vi "MeanData.vi"(11 "Prop in":T1[](array[typedef])) -> (3 "Poperties out":T1={"Raw Data"=[[0.0], [0.0234375], [0.9609375]], "Poperties"={"RMS values"=[], "Max"=[], "Min"=[], "A(8)"=[], "t"=0.0, "A(8) Axis"=0.0, "Aw"=[], "Ak 30min"=0.0, "Ak_axis"=0, "Spec"=[]}, "Power Spectrum / PSD"=[]})   [LabVIEW 2019]
uses:
  Communication/TypeDef/#TypeDef_PropGraph.ctl
  Communication/TypeDef/#TypeDef_PropertiesToSave.ctl
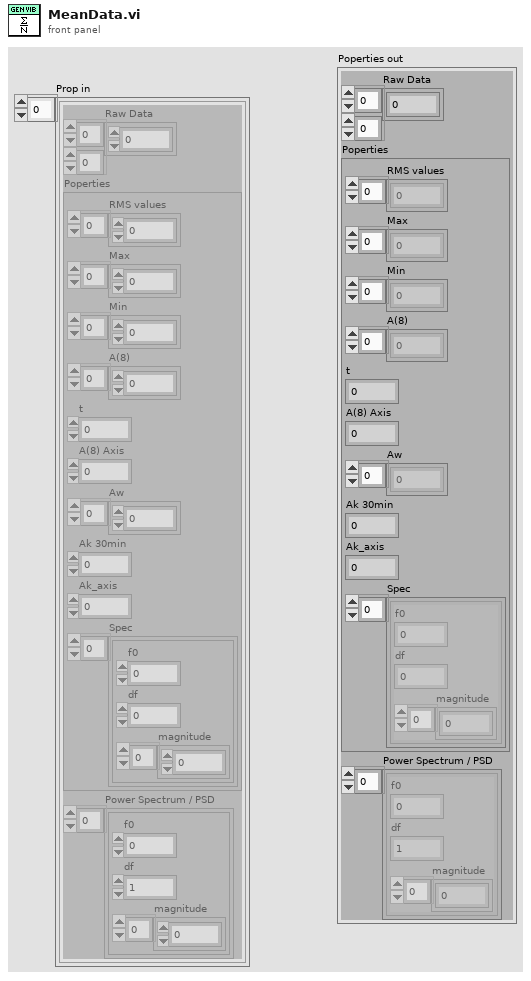
[diagram p1: front panel]
types:
  T1 = typedef "#TypeDef_PropGraph.ctl" = cluster{"Raw Data":dbl[][], "Poperties":T2, "Power Spectrum / PSD":cluster{"f0":dbl, "df":dbl, "magnitude":dbl[]}[]}
  T2 = typedef "#TypeDef_PropertiesToSave.ctl" = cluster{"RMS values":dbl[], "Max":dbl[], "Min":dbl[], "A(8)":dbl[], "t":dbl, "A(8) Axis":dbl, "Aw":dbl[], "Ak 30min":dbl, "Ak_axis":i32, "Spec":cluster{"f0":dbl, "df":dbl, "magnitude":dbl[]}[]}
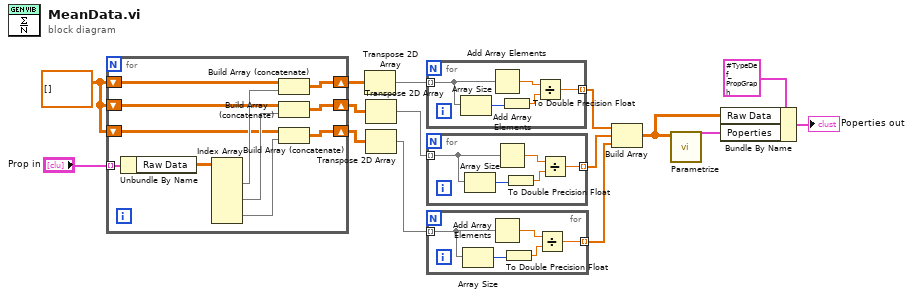
[diagram p0: block diagram]
diagram:
  w6 = dbl[][] []
  n1 = for {
    tunnel: "Prop in" -> [w26] mode=indexing
    shift-right: [w25] -> w7
    shift-left: w6 -> [w24]
    shift-right: [w20] -> w9
    shift-left: w6 -> [w19]
    shift-right: [w17] -> w11
    shift-left: w6 -> [w16]
    n2 = Unbundle By Name(w26) -> ("Raw Data"=w23:dbl[][])
    n3 = Index Array(array=w23) -> (element #1=w22:dbl[], element #2=w21:dbl[], element #3=w18:dbl[])  [unwired: 6 in]
    n4 = Build Array (concatenate)(w24, w22) -> (w25:dbl[][])
    n5 = Build Array (concatenate)(w19, w21) -> (w20:dbl[][])
    n6 = Build Array (concatenate)(w16, w18) -> (w17:dbl[][])
  }
  n7 = Transpose 2D Array(2D array=w7) -> (transposed array=w8:dbl[][])
  n8 = Transpose 2D Array(2D array=w9) -> (transposed array=w10:dbl[][])
  n9 = Transpose 2D Array(2D array=w11) -> (transposed array=w12:dbl[][])
  n10 = for {
    tunnel: w8 -> [w31] mode=indexing
    tunnel: [w30] -> w13 mode=indexing
    n11 = Array Size(array=w31) -> (size(s)=w29:i32)
    n12 = Add Array Elements(numeric array=w31) -> (sum=w28:dbl)
    n13 = To Double Precision Float(number=w29) -> (double precision float=w27:dbl)
    n14 = Divide(x=w28, y=w27) -> (x/y=w30:dbl)
  }
  n15 = for {
    tunnel: w10 -> [w36] mode=indexing
    tunnel: [w35] -> w14 mode=indexing
    n16 = Array Size(array=w36) -> (size(s)=w34:i32)
    n17 = Add Array Elements(numeric array=w36) -> (sum=w33:dbl)
    n18 = To Double Precision Float(number=w34) -> (double precision float=w32:dbl)
    n19 = Divide(x=w33, y=w32) -> (x/y=w35:dbl)
  }
  n20 = for {
    tunnel: w12 -> [w41] mode=indexing
    tunnel: [w40] -> w15 mode=indexing
    n21 = Array Size(array=w41) -> (size(s)=w39:i32)
    n22 = Add Array Elements(numeric array=w41) -> (sum=w38:dbl)
    n23 = To Double Precision Float(number=w39) -> (double precision float=w37:dbl)
    n24 = Divide(x=w38, y=w37) -> (x/y=w40:dbl)
  }
  n25 = Build Array(w13, w14, w15) -> (w3:dbl[][])
  n26 = call "Parametrize.vi"("Raw Data"=w3) -> ("Poperties"=w2:T2)  [unwired: 10 in]
  n27 = Bundle By Name(cluster=T1 {"Raw Data"=[[0.0], [0.0234375], [0.9609375]], "Poperties"={"RMS values"=[], "Max"=[], "Min"=[], "A(8)"=[], "t"=0.0, "A(8) Axis"=0.0, "Aw"=[], "Ak 30min"=0.0, "Ak_axis"=0, "Spec"=[]}, "Power Spectrum / PSD"=[]} ("Prop out"), "Raw Data"=w3, "Poperties"=w2) -> (→"Poperties out":T1)
